vi "UHR-Fleezers Control (host) -TL FB Corrected Ronen semipassive - stepping.vi"(0 "Tab Control":T5(tab)=enum."Trap Control (RF)") -> ()   [LabVIEW 2013] (continued)
        n1835 = Build Array (concatenate)(w2860, w2859) -> (w2841:dbl[])
        n1836 = feedback #13(w2764) -> (w2766:dbl[])
        n1837 = Build Array (concatenate)(w2766, w2764) -> (w2765:dbl[])
        n1838 = local read "Scan steps (MCL)"() -> (w2746:u64)
        n1839 = Select(t=w2859, s=w2763, f=w2841) -> (s? t:f=w2845:dbl[])
        n1840 = feedback-in #12(w2845) -> ()
        n1841 = Select(t=w2764, s=w2763, f=w2765) -> (s? t:f=w2747:dbl[])
        n1842 = feedback-in #13(w2747) -> ()
        n1843 = local read "Scan lines (y)"() -> (w2732:u64)
        n1844 = local read "N APD Samp/step"() -> (w2748:dbl)
        n1845 = feedback #14(w2790) -> (w2847:dbl[])
        n1846 = Build Array (concatenate)(w2847, w2790) -> (w2838:dbl[])
        n1847 = feedback #15(w2797) -> (w2857:dbl[])
        n1848 = Build Array (concatenate)(w2857, w2797) -> (w2856:dbl[])
        n1849 = feedback #16(w2792) -> (w2849:dbl[])
        n1850 = Build Array (concatenate)(w2849, w2792) -> (w2850:dbl[])
        n1851 = Select(t=w2790, s=w2763, f=w2838) -> (s? t:f=w2794:dbl[])
        n1852 = feedback-in #14(w2794) -> ()
        n1853 = Select(t=w2797, s=w2763, f=w2856) -> (s? t:f=w2796:dbl[])
        n1854 = feedback-in #15(w2796) -> ()
        n1855 = Select(t=w2792, s=w2763, f=w2850) -> (s? t:f=w2795:dbl[])
        n1856 = feedback-in #16(w2795) -> ()
        n1857 = Multiply(x=w2746, y=u64 2) -> (x*y=w2731:u64)
        n1858 = call "integrate 1D array interval - double.vi"("Ave N"=w2748, "Array In"=w2747) -> ("Array Out"=w2759:dbl[])  [unwired: 1 out]
        n1859 = call "integrate 1D array interval - double.vi"("Ave N"=w2748, "Array In"=w2845) -> ("Array Out"=w2844:dbl[])  [unwired: 1 out]
        n1860 = Array Size(array=w2759) -> (size(s)=w2760:i32)
        n1861 = Array Size(array=w2844) -> (size(s)=w2846:i32)
        n1862 = Multiply(x=w2732, y=w2731) -> (x*y=w2762:u64)
        n1863 = Multiply(x=w2732, y=w2731) -> (x*y=w2854:u64)
        n1864 = call-poly <vilib>:"Mean.vi"("X"=w2794) -> ("mean"=w2778:dbl)  [unwired: 1 out]
        n1865 = Subtract(x=w2762, y=w2760) -> (x-y=w2753:u64)
        n1866 = call-poly <vilib>:"Mean.vi"("X"=w2796) -> ("mean"=w2783:dbl)  [unwired: 1 out]
        n1867 = call-poly <vilib>:"Mean.vi"("X"=w2795) -> ("mean"=w2781:dbl)  [unwired: 1 out]
        n1868 = call-poly <vilib>:"Mean.vi"("X"=w2759) -> ("mean"=w2750:dbl)  [unwired: 1 out]
        n1869 = Subtract(x=w2854, y=w2846) -> (x-y=w2788:u64)
        n1870 = call-poly <vilib>:"Mean.vi"("X"=w2844) -> ("mean"=w2785:dbl)  [unwired: 1 out]
        n1871 = Initialize Array(1.0 ("element"), w2753) -> (w2749:dbl[])
        n1872 = Initialize Array(1.0 ("element"), w2788) -> (w2779:dbl[])
        n1873 = Multiply(x=w2749, y=w2750) -> (x*y=w2751:dbl[])
        n1874 = Multiply(x=w2779, y=w2781) -> (x*y=w2782:dbl[])
        n1875 = Multiply(x=w2779, y=w2783) -> (x*y=w2784:dbl[])
        n1876 = Multiply(x=w2779, y=w2778) -> (x*y=w2780:dbl[])
        n1877 = Multiply(x=w2779, y=w2785) -> (x*y=w2786:dbl[])
        n1878 = Build Array (concatenate)(w2794, w2780) -> (w2848:dbl[])
        n1879 = Build Array (concatenate)(w2796, w2784) -> (w2852:dbl[])
        n1880 = Build Array (concatenate)(w2795, w2782) -> (w2851:dbl[])
        n1881 = Build Array (concatenate)(w2759, w2751) -> (w2761:dbl[])
        n1882 = Build Array (concatenate)(w2844, w2786) -> (w2853:dbl[])
        n1883 = Reshape Array(w2848, w2732, w2731) -> (w2814:dbl[][])
        n1884 = Reshape Array(w2761, w2732, w2731) -> (w2757:dbl[][])
        n1885 = Reshape Array(w2852, w2732, w2731) -> (w2806:dbl[][])
        n1886 = Reshape Array(w2851, w2732, w2731) -> (w2821:dbl[][])
        n1887 = Reshape Array(w2853, w2732, w2731) -> (w2831:dbl[][])
        n1888 = Array Subset(array=w2821, index (col)=0 ("index"), length (col)=w2746) -> (w2826:dbl[][])  [unwired: 2 in]
        n1889 = Array Subset(array=w2821, index (col)=w2746) -> (w2824:dbl[][])  [unwired: 3 in]
        n1890 = Array Subset(array=w2806, index (col)=0 ("index"), length (col)=w2746) -> (w2812:dbl[][])  [unwired: 2 in]
        n1891 = Array Subset(array=w2806, index (col)=w2746) -> (w2810:dbl[][])  [unwired: 3 in]
        n1892 = Array Subset(array=w2757, index (col)=0 ("index"), length (col)=w2746) -> (w2756:dbl[][])  [unwired: 2 in]
        n1893 = Array Subset(array=w2757, index (col)=w2746) -> (w2754:dbl[][])  [unwired: 3 in]
        n1894 = Array Subset(array=w2831, index (col)=0 ("index"), length (col)=w2746) -> (w2830:dbl[][])  [unwired: 2 in]
        n1895 = Array Subset(array=w2831, index (col)=w2746) -> (w2828:dbl[][])  [unwired: 3 in]
        n1896 = Array Subset(array=w2814, index (col)=0 ("index"), length (col)=w2746) -> (w2819:dbl[][])  [unwired: 2 in]
        n1897 = Array Subset(array=w2814, index (col)=w2746) -> (w2817:dbl[][])  [unwired: 3 in]
        n1898 = for {
          tunnel: w2826 -> [w2868] mode=indexing
          tunnel: [w2867] -> w2825 mode=indexing
          workers-P: _ -> [_]
          n1899 = Reverse 1D Array(array=w2868) -> (reversed array=w2867:dbl[])
        }
        n1900 = for {
          tunnel: w2812 -> [w2864] mode=indexing
          tunnel: [w2863] -> w2811 mode=indexing
          workers-P: _ -> [_]
          n1901 = Reverse 1D Array(array=w2864) -> (reversed array=w2863:dbl[])
        }
        n1902 = for {
          tunnel: w2756 -> [w2862] mode=indexing
          tunnel: [w2861] -> w2755 mode=indexing
          workers-P: _ -> [_]
          n1903 = Reverse 1D Array(array=w2862) -> (reversed array=w2861:dbl[])
        }
        n1904 = for {
          tunnel: w2830 -> [w2870] mode=indexing
          tunnel: [w2869] -> w2829 mode=indexing
          workers-P: _ -> [_]
          n1905 = Reverse 1D Array(array=w2870) -> (reversed array=w2869:dbl[])
        }
        n1906 = for {
          tunnel: w2819 -> [w2866] mode=indexing
          tunnel: [w2865] -> w2818 mode=indexing
          workers-P: _ -> [_]
          n1907 = Reverse 1D Array(array=w2866) -> (reversed array=w2865:dbl[])
        }
        n1908 = Index Array(array=w2831, index (row)=0) -> (element=→"Waveform Graph":dbl[])  [unwired: 1 in]
        n1909 = Add(x=w2825, y=w2824) -> (x+y=w2823:dbl[][])
        n1910 = Add(x=w2811, y=w2810) -> (x+y=w2809:dbl[][])
        n1911 = Add(x=w2755, y=w2754) -> (x+y=w2739:dbl[][])
        n1912 = Add(x=w2829, y=w2828) -> (x+y=w2803:dbl[][])
        n1913 = Add(x=w2818, y=w2817) -> (x+y=w2816:dbl[][])
        n1914 = Divide(x=w2809, y=2) -> (x/y=w2807:dbl[][])
        n1915 = Divide(x=w2823, y=2) -> (x/y=w2768:dbl[][])
        n1916 = Divide(x=w2816, y=2) -> (x/y=w2770:dbl[][])
        n1917 = To Single Precision Float(number=w2803) -> (single precision float=w2802:sgl[][])
        n1918 = Transpose 2D Array(2D array=w2807) -> (transposed array=→"Data map":dbl[][])
        n1919 = To Single Precision Float(number=w2739) -> (single precision float=w2743:sgl[][])
        n1920 = To Single Precision Float(number=w2768) -> (single precision float=w2774:sgl[][])
        n1921 = To Single Precision Float(number=w2770) -> (single precision float=w2771:sgl[][])
        n1922 = call "IMAQ ArrayToImage"("Image Pixels (Float)"=w2802, "Image"=w2736) -> ("Image Out"=w2805:T3)  [unwired: 8 in, 1 out]
        n1923 = call "IMAQ ArrayToImage"("Image Pixels (Float)"=w2743, "Image"=w2735) -> ("Image Out"=w2745:T3)  [unwired: 8 in, 1 out]
        n1924 = call "IMAQ ArrayToImage"("Image Pixels (Float)"=w2774, "Image"=w2734) -> ("Image Out"=w2776:T3)  [unwired: 8 in, 1 out]
        n1925 = call "IMAQ ArrayToImage"("Image Pixels (Float)"=w2771, "Image"=w2733) -> ("Image Out"=w2773:T3)  [unwired: 8 in, 1 out]
        n1926 = call "IMAQ Symmetry"("Type of Symmetry"=w2804, "Image Src"=w2805) -> ("Image Dst Out"=w2800:T3)  [unwired: 3 in, 1 out]
        n1927 = call "IMAQ Symmetry"("Type of Symmetry"=w2744, "Image Src"=w2745) -> ("Image Dst Out"=w2741:T3)  [unwired: 3 in, 1 out]
        n1928 = call "IMAQ Symmetry"("Type of Symmetry"=w2775, "Image Src"=w2776) -> ("Image Dst Out"=→"Detection Laser X":T3)  [unwired: 3 in, 1 out]
        n1929 = call "IMAQ Symmetry"("Type of Symmetry"=w2772, "Image Src"=w2773) -> ("Image Dst Out"=→"Detection Laser Y":T3)  [unwired: 3 in, 1 out]
        n1930 = call "IMAQ Set Simple Calibration"("Calibration Axis Info"=T37 {"Origin Pixel"={"X"=0.0, "Y"=0.0}, "Angle Relative to Horizontal (deg)"=0.0, "Axis Reference"=0}, "Grid Descriptor"=T38 {"X Step"=0.3, "Y Step"=0.3, "Unit"=enum."Undefined"}, "Image"=w2800) -> ("Calibrated Image"=→"APD 1":T3)  [unwired: 7 in, 1 out]
        n1931 = call "IMAQ Set Simple Calibration"("Calibration Axis Info"=T37 {"Origin Pixel"={"X"=0.0, "Y"=0.0}, "Angle Relative to Horizontal (deg)"=0.0, "Axis Reference"=0}, "Grid Descriptor"=T38 {"X Step"=0.3, "Y Step"=0.3, "Unit"=enum."Undefined"}, "Image"=w2741) -> ("Calibrated Image"=→"APD 2":T3)  [unwired: 7 in, 1 out]
      }
    }
    n1932 = Subtract(x=w2283, y="APD 2 Offset") -> (x-y=w2280:waveform(dbl))
    n1933 = Subtract(x=w2285, y="APD 1 Offset") -> (x-y=w2281:waveform(dbl))
    n1934 = Index Array(array=w2300, index=3) -> (element=w2367:waveform(dbl))
    n1935 = Index Array(array=w2300, index=6) -> (element=w2364:waveform(dbl))
    n1936 = Build Array(w2281, w2280) -> (→"APD Chart":waveform(dbl)[])
    n1937 = Array Size(array=w2357) -> (size(s)=w2407:i32)
    n1938 = call <vilib>:"Std Deviation and Variance.vi"("X"=w2293) -> ("standard deviation"=w2292:dbl)  [unwired: 1 in, 2 out]
    n1939 = Add Array Elements(numeric array=w2293) -> (sum=w2295:u32)
    n1940 = Add Array Elements(numeric array=w2357) -> (sum=w2417:u32)
    n1941 = call <vilib>:"Std Deviation and Variance.vi"("X"=w2357) -> ("standard deviation"=w2356:dbl)  [unwired: 1 in, 2 out]
    n1942 = Divide(x=w2292, y=w2291) -> (x/y=w2288:dbl)
    "Rate sigma (Hz) 2" <- w2288
    n1943 = Multiply(x=w2291, y=w2407) -> (x*y=w2294:dbl)
    "Int. Time (s)" <- w2294
    n1944 = Divide(x=w2295, y=w2294) -> (x/y=w2289:dbl)
    "APD 2 Rate (Hz)" <- w2289
    n1945 = Divide(x=w2417, y=w2294) -> (x/y=w2354:dbl)
    "APD 1 Rate (Hz)" <- w2354
    n1946 = Divide(x=w2356, y=w2291) -> (x/y=w2355:dbl)
    "Rate sigma (Hz)" <- w2355
    n1947 = Divide(x=w2288, y=w2289) -> (x/y=→"Sigma/Mean 2":dbl)
    n1948 = Divide(x=w2355, y=w2354) -> (x/y=→"Sigma/Mean":dbl)
    n1949 = case shown="2" "Calibration" {
      tunnel: "T1 alpha_x (nm/V)" -> [_ w2699 w2720]
      tunnel: "T1 kappa_x (pN/nm)" -> [_ _ w2710]
      tunnel: "T2 alpha_x (nm/V)" -> [_ w2698 w2718]
      tunnel: "T2 kappa_x (pN/nm)" -> [_ _ w2711]
      tunnel: w2367 -> [w2681 w2696 w2716]
      tunnel: w2364 -> [w2680 w2694 w2714]
      tunnel: [w2681 w2693 w2713] -> w2393
      tunnel: [w2680 w2692 w2712] -> w2392
      tunnel: ["T1 X (V)" ("Label.Text") "T1 X (nm)" ("Label.Text") "T1 X (pN)" ("Label.Text")] -> w2385
      tunnel: ["T2 X (V)" ("Label.Text") "T2 X (nm)" ("Label.Text") "T2 X (pN)" ("Label.Text")] -> w2384
      tunnel: ["Position (V)" ("Label.Text") "Position (nm)" ("Label.Text") "Force (pN)" ("Label.Text")] -> w2386
      tunnel: w2366 -> [_ w2684 w2703]
      tunnel: w2368 -> [_ w2687 w2705]
      tunnel: ["Mean (V)" ("Label.Text") "Mean (nm)" ("Label.Text") "Mean (pN)" ("Label.Text")] -> w2381
      tunnel: ["Difference (V)" ("Label.Text") "Difference (nm)" ("Label.Text") "Difference (pN)" ("Label.Text")] -> w2308
      frame 0, Default {
      }
      frame 1 {
        # "position"
        n1950 = Unbundle By Name(w2696) -> ("Y"=w2700:dbl[])
        n1951 = Unbundle By Name(w2694) -> ("Y"=w2685:dbl[])
        n1952 = Subtract(x=w2700, y=w2687) -> (x-y=w2688:dbl[])
        n1953 = Subtract(x=w2685, y=w2684) -> (x-y=w2686:dbl[])
        n1954 = Multiply(x=w2686, y=w2698) -> (x*y=w2695:dbl[])
        n1955 = Multiply(x=w2699, y=w2688) -> (x*y=w2697:dbl[])
        n1956 = Bundle By Name(cluster=w2694, "Y"=w2695) -> (w2692:waveform(dbl))
        n1957 = Bundle By Name(cluster=w2696, "Y"=w2697) -> (w2693:waveform(dbl))
      }
      frame 2 {
        # "force"
        n1958 = Unbundle By Name(w2716) -> ("Y"=w2721:dbl[])
        n1959 = Unbundle By Name(w2714) -> ("Y"=w2719:dbl[])
        n1960 = Subtract(x=w2719, y=w2703) -> (x-y=w2704:dbl[])
        n1961 = Subtract(x=w2721, y=w2705) -> (x-y=w2706:dbl[])
        n1962 = Compound Arithmetic op=MULTIPLY(w2704, w2718, w2711) -> (w2715:dbl[])
        n1963 = Compound Arithmetic op=MULTIPLY(w2710, w2720, w2706) -> (w2717:dbl[])
        n1964 = Bundle By Name(cluster=w2714, "Y"=w2715) -> (w2712:waveform(dbl))
        n1965 = Bundle By Name(cluster=w2716, "Y"=w2717) -> (w2713:waveform(dbl))
      }
    }
    n1966 = feedback-in #17("Calibration") -> ()
    n1967 = feedback #17(u16 1 ("Calibration")) -> (w2388:u16)
    n1968 = local read "Trap 2 Bead Size (nm)"() -> (w2188:dbl)
    n1969 = local read "Trap 1 Bead Size (nm)"() -> (w2187:dbl)
    n1970 = local read "AOM X Cal (nm/MHz)"() -> (w2185:dbl)
    n1971 = local read "Trap Delta (MHz)"() -> (w2184:dbl)
    n1972 = Not Equal?(x=w2388, y="Calibration") -> (x != y?=w2345:bool)
    n1973 = Multiply(x=w2185, y=w2184) -> (x*y=w2189:dbl)
    n1974 = Add(x=w2188, y=w2187) -> (x+y=w2191:dbl)
    n1975 = Unbundle By Name(w2367) -> ("Y"=w2370:dbl[])
    n1976 = Unbundle By Name(w2364) -> ("Y"=w2373:dbl[])
    n1977 = Divide(x=w2191, y=2.0) -> (x/y=w2186:dbl)
    n1978 = Subtract(x=w2370, y=w2368) -> (x-y=w2371:dbl[])
    n1979 = Subtract(x=w2373, y=w2366) -> (x-y=w2372:dbl[])
    n1980 = disable-structure shown="Enabled" {
      disable-tunnel: [-1.0 ("y") 1.0] -> w2374
      frame Disabled {
      }
      frame Enabled {
      }
    }
    n1981 = Multiply(x=w2372, y="T2 alpha_x (nm/V)") -> (x*y=w2363:dbl[])
    n1982 = Multiply(x="T1 alpha_x (nm/V)", y=w2371) -> (x*y=w2362:dbl[])
    n1983 = Multiply(x=w2392, y=w2374) -> (x*y=w2375:waveform(dbl))
    n1984 = case shown="False" "Read Lateness and Rel Phase" {
      tunnel: w2161 -> [w2647 w2669]
      tunnel: w2200 -> [w2648 w2668]
      tunnel: [w2647 w2667] -> w2360
      tunnel: [w2648 w2666] -> w2359
      frame False {
      }
      frame True {
        n1985 = xnode "Read/Write Control"("FPGA VI Reference In"=w2669, "error in"=w2668) -> ("FPGA VI Reference Out"=w2667:T20, "error out"=w2666:errorcluster, "GI Relative phase"=→"GI relative phase":i16, "Relative phase"=→"Relative phase (AI1)":i16, "AI Late Counter"=→"Late Counter (AI1)":u8, "GI Late Counter"=→"GI Late Counter":u8, "MCL Late Counter"=→"MCL Late Counter":u8, "MCL Relative Phase"=→"Relative Phase (MCL)":i16, "APD Acq Relative Phase"=→"APD Acq Relative Phase":i16, "APD 1 Gate Relative Phase"=→"APD 1 Gate Relative Phase":i16, "APD 2 Gate Relative Phase"=→"APD 2 Gate Relative Phase":i16, "APD Acq Late Counter"=→"APD Acq Late Counter":u16, "APD 1 Gate Late Counter"=→"APD 1 Gate Late Counter":u8, "APD 2 Gate Late Counter"=→"APD 2 Gate Late Counter":u8, "Green FB Relative Phase"=→"Relative phase (Green FB)":i16, "GI Relative phase 2"=→"GI relative phase 2":i16, "GI Late Counter 2"=→"GI Late Counter 2":u16, "Trap Pos FIFO Timeout"=→"Trap Pos FIFO Timeout":u16, "Trap AI FIFO Timeout"=→"Trap AI FIFO Timeout":u16)
      }
    }
    n1986 = Subtract(x=w2363, y=w2362) -> (x-y=w2183:dbl[])
    n1987 = call-poly <vilib>:"Mean.vi"("X"=w2183) -> ("mean"=w2190:dbl)  [unwired: 1 out]
    n1988 = Add(x=w2189, y=w2190) -> (x+y=w2193:dbl)
    n1989 = Subtract(x=w2193, y=w2186) -> (x-y=→"Tether Extension (nm, calculated)":dbl)
    n1990 = Unbundle By Name(w2392) -> ("Y"=w2333:dbl[])
    n1991 = Unbundle By Name(w2393) -> ("Y"=w2334:dbl[])
    n1992 = Build Array(w2393, w2375) -> (→"Force":waveform(dbl)[])
    n1993 = Subtract(x=w2183, y="Offset (nm)") -> (x-y=w2331:dbl[])
    n1994 = call-poly <vilib>:"Mean.vi"("X"=w2333) -> ("mean"=w2312:dbl)  [unwired: 1 out]
    "T2 X" <- w2312
    n1995 = Absolute Value(x=w2334) -> (abs(x)=w2335:dbl[])
    n1996 = Absolute Value(x=w2333) -> (abs(x)=w2336:dbl[])
    n1997 = call-poly <vilib>:"Mean.vi"("X"=w2334) -> ("mean"=w2313:dbl)  [unwired: 1 out]
    "T1 X" <- w2313
    n1998 = Add(x=w2335, y=w2336) -> (x+y=w2337:dbl[])
    n1999 = Bundle By Name(cluster=w2367, "Y"=w2331) -> (w2299:waveform(dbl))
    "Bead Separation" <- w2299
    n2000 = Divide(x=w2337, y=2.0) -> (x/y=→"Vec Mean of T1 T2":dbl[])
    n2001 = case shown="True" w2345 {
      tunnel: w2386 -> [_ w2674]
      tunnel: w2385 -> [_ w2673]
      tunnel: w2384 -> [_ w2672]
      tunnel: w2381 -> [_ w2671]
      tunnel: w2308 -> [_ w2670]
      frame False {
      }
      frame True {
        n2002 = property on="Force" class="WFChart (strict)"("YScale.NameLbl.Text"=w2674) -> ()  [unwired: 2 in, 2 out]
        n2003 = property on="T2 X" class="DigNum (strict)"("Caption.Text"=w2672) -> ()  [unwired: 2 in, 2 out]
        n2004 = property on="T1 X" class="DigNum (strict)"("Caption.Text"=w2673) -> ()  [unwired: 2 in, 2 out]
        n2005 = property on="Mean" class="DigNum (strict)"("Caption.Text"=w2671) -> ()  [unwired: 2 in, 2 out]
        n2006 = property on="Difference" class="DigNum (strict)"("Caption.Text"=w2670) -> ()  [unwired: 2 in, 2 out]
      }
    }
    n2007 = local read "Tether"() -> (w2339:bool)
    n2008 = Absolute Value(x=w2313) -> (abs(x)=w2310:dbl)
    n2009 = Absolute Value(x=w2312) -> (abs(x)=w2309:dbl)
    n2010 = Add(x=w2310, y=w2309) -> (x+y=w2383:dbl)
    n2011 = Subtract(x=w2310, y=w2309) -> (x-y=→"Difference":dbl)
    n2012 = feedback #18(w2331) -> (w2330:dbl[])
    n2013 = Divide(x=w2383, y=2.0) -> (x/y=w2158:dbl)
    "Mean" <- w2158
    n2014 = case shown="True" w2339 {
      tunnel: w2158 -> [_ w2606]
      frame False {
      }
      frame True {
        n2015 = Greater?(x="Lost Tether Alarm Threshold (pN)", y=w2606) -> (0:w2604:bool)
        n2016 = case shown="True" w2604 {
          frame False {
          }
          frame True {
            n2017 = flat-sequence {
              frame #0 {
                # "stop only if saving"
                n2018 = local read "Saving..."() -> (w2619:bool)
                n2019 = And(x=w2619, y="TA Cancel Save?") -> (x .and. y?=w2618:bool)
                n2020 = local write "Stop Saving"(w2618) -> ()
              }
              frame #1 {
                n2021 = case shown="True" "TA Green Off?" {
                  frame False {
                  }
                  frame True {
                    w2622 = FALSE ("Fl. Triggered...")
                    n2022 = local write "Fl. Triggered..."(w2622) -> ()
                    n2023 = property on="Green Laser ON/Interlacing" class="Bool (strict)"("Val(Sgnl)"=w2622) -> ()  [unwired: 2 in, 2 out]
                  }
                }
              }
            }
            n2024 = local read "Time tether formed"() -> (w2613:timestamp)
            n2025 = Get Date/Time In Seconds() -> (seconds since 1Jan1904=w2614:timestamp)
            n2026 = Subtract(x=w2614, y=w2613) -> (x-y=w2612:dbl)
            n2027 = Number To Decimal String(number=w2612) -> (decimal integer string=w2609:string)  [unwired: 1 out]
            n2028 = local read "Messages"() -> (w2616:string)
            n2029 = call <vilib>:"Beep.vi"() -> ()  [unwired: 3 in, 9 out]
            n2030 = Concatenate Strings("Lost tether (" ("Message to add"), w2609, " s)." ("string")) -> (w2611:string)
            n2031 = local write "Tether"(FALSE ("Tether")) -> ()
            n2032 = call "Update messages.vi"("Message to add"=w2611, "Old message string"=w2616) -> ("New message string"=w2615:string)
            n2033 = local write "Messages"(w2615) -> ()
            n2034 = property on="Trap Pos. FB ON" class="Bool (strict)"("Val(Sgnl)"=FALSE ("Value (Signaling)")) -> ()  [unwired: 2 in, 2 out]
          }
        }
      }
    }
    n2035 = Build Array (concatenate)(w2331, w2330) -> (w2329:dbl[])
    n2036 = Split 1D Array(array=w2329, index=w2211) -> (first subarray=w2325:dbl[])  [unwired: 1 out]
    n2037 = feedback-in #18(w2325) -> ()
    n2038 = call-poly <vilib>:"Mean.vi"("X"=w2325) -> ("mean"=w2324:dbl)  [unwired: 1 out]
    "Bead Mean (nm)" <- w2324
    n2039 = Subtract(x=w2325, y=w2324) -> (x-y=w2323:dbl[])
    n2040 = Square(x=w2323) -> (x^2=w2322:dbl[])
    n2041 = case shown="True" "Semi Passive ON" {
      tunnel: "Semi Passive mode" -> [_ w2485]
      tunnel: "Jump Force (pN)" -> [_ w2484]
      tunnel: w2158 -> [_ w2483]
      frame False {
      }
      frame True {
        n2042 = case shown="\"Use Feedback\"" w2485 {
          tunnel: w2484 -> [_ w2488 w2504]
          tunnel: w2483 -> [_ w2487 w2503]
          frame "None" {
          }
          frame "Use Feedback" {
            n2043 = local read "Target Force (pN)"() -> (w2490:dbl)
            n2044 = Less?(x=w2488, y=w2490) -> (x < y?=w2489:bool)
            n2045 = case shown="True" w2489 {
              tunnel: w2488 -> [w2497 w2500]
              tunnel: w2487 -> [w2496 w2499]
              tunnel: [w2495 w2498] -> w2486
              frame False {
                n2046 = Less?(x=w2497, y=w2496) -> (x < y?=w2495:bool)
              }
              frame True {
                n2047 = Greater?(x=w2500, y=w2499) -> (0:w2498:bool)
              }
            }
            n2048 = case shown="True" w2486 {
              frame False {
                n2049 = local read "Trap Pos. FB ON"() -> (w2491:bool)
                n2050 = case shown="True" w2491 {
                  frame False {
                  }
                  frame True {
                    n2051 = property on="Trap Pos. FB ON" class="Bool (strict)"("Val(Sgnl)"=FALSE) -> ()  [unwired: 2 in, 2 out]
                  }
                }
              }
              frame True {
                n2052 = local read "Trap Pos. FB ON"() -> (w2493:bool)
                n2053 = case shown="False" w2493 {
                  frame False {
                    n2054 = property on="Trap Pos. FB ON" class="Bool (strict)"("Val(Sgnl)"=TRUE) -> ()  [unwired: 2 in, 2 out]
                  }
                  frame True {
                  }
                }
              }
            }
          }
          frame "Sharp Jump" {
            n2055 = local read "Target Force (pN)"() -> (w2506:dbl)
            n2056 = Greater?(x=w2504, y=w2506) -> (0:w2505:bool)
            n2057 = case shown="True" w2505 {
              tunnel: w2504 -> [w2521 w2525]
              tunnel: w2503 -> [w2522 w2524]
              tunnel: [w2520 w2523] -> w2502
              frame False {
                n2058 = Greater?(x=w2522, y=w2521) -> (0:w2520:bool)
              }
              frame True {
                n2059 = Less?(x=w2525, y=w2524) -> (x < y?=w2523:bool)
              }
            }
            n2060 = Subtract(x=w2504, y=w2506) -> (x-y=w2501:dbl)
            n2061 = case shown="True" w2502 {
              tunnel: w2501 -> [_ w2512]
              frame False {
              }
              frame True {
                n2062 = local read "T1 kappa_x (pN/nm)"() -> (w2517:dbl)
                n2063 = local read "T2 kappa_x (pN/nm)"() -> (w2518:dbl)
                n2064 = Reciprocal(x="DNA stiffness (pN / nm)") -> (1/x=w2514:dbl)
                n2065 = Reciprocal(x=w2517) -> (1/x=w2516:dbl)
                n2066 = Reciprocal(x=w2518) -> (1/x=w2515:dbl)
                n2067 = Compound Arithmetic op=ADD(w2516, w2515, w2514) -> (w2513:dbl)
                n2068 = local read "AOM X Cal (nm/MHz)"() -> (w2511:dbl)
                n2069 = Multiply(x=w2513, y=w2512) -> (x*y=w2510:dbl)
                n2070 = local read "Trap Delta (MHz)"() -> (w2508:dbl)
                n2071 = Divide(x=w2510, y=w2511) -> (x/y=w2509:dbl)
                n2072 = Subtract(x=w2508, y=w2509) -> (x-y=w2507:dbl)
                n2073 = property on="Trap Delta (MHz)" class="DigNum (strict)"("Val(Sgnl)"=w2507) -> ()  [unwired: 2 in, 2 out]
              }
            }
          }
        }
      }
    }
    n2074 = call-poly <vilib>:"Mean.vi"("X"=w2322) -> ("mean"=w2321:dbl)  [unwired: 1 out]
    n2075 = Square Root(x=w2321) -> (sqrt(x)=w2320:dbl)
    n2076 = Multiply(x=10.0, y=w2320) -> (x*y=→"RMS (Ang)":dbl)
    n2077 = xnode "Read/Write Control"("FPGA VI Reference In"=w2360, "error in"=w2359) -> ("FPGA VI Reference Out"=w2471:T20, "error out"=w2465:errorcluster, "AI4 Y Sum Set 1"=w2461, "AI4 Y Sum Set 2"=w2460, "AI1 X Set 1"=w2245:fxp<+/-,16,1>, "AI1 X Set 2"=w2244:fxp<+/-,16,1>, "Trap Pos FB Int Signal"=→"Trap Pos FB Int Signal":fxp<+/-,24,9>, "Trap Pos FB Int-Norm Signal"=→"Trap Pos FB Int-Norm Signal":fxp<+/-,16,1>, "Trap Pos FB Action"=w2238:i64, "Scanning"=→"AOD Scanning":bool, "Scan I"=→"AOD Scan I":u64, "Scanning MCL"=w2463:bool, "Scan I (MCL)"=→"MCL Scan I":u64, "Green FB Signals"=w2402:T48)  [unwired: 1 out]
    "MCL Scanning" <- w2463
    "Trap Pos FB Action" <- w2238
    n2078 = local read "AI2 (V)"() -> (w2462:cluster{"Set 1":dbl, "Set 2":dbl})
    n2079 = Bundle By Name(cluster=w2462, "Set 1"=w2461, "Set 2"=w2460) -> (w2458:cluster{"Set 1":dbl, "Set 2":dbl})
    n2080 = Divide(x=w2238, y=327.67) -> (x/y=→"Action (%)":dbl)
    n2081 = local read "Trap X (AI1)"() -> (w2258:T1)
    n2082 = Divide(x=w2458, y=3276.7) -> (x/y=w2457:cluster{"Set 1":dbl, "Set 2":dbl})
    n2083 = local write "AI2 (V)"(w2457) -> ()
    n2084 = Bundle(cluster=w2258, "Trap 1"=w2245, "Trap 2"=w2244) -> (→"Trap X (AI1)":T1)
    n2085 = Divide(x=w2402, y=3276.7) -> (x/y=w2398:T49)
    n2086 = Unbundle By Name(w2398) -> ("Green FB Ch 0"=w2401:dbl, "Green FB Ch 1"=w2400:dbl, "Green FB Ch 2"=w2399:dbl)
    n2087 = Divide(x=w2401, y=w2399) -> (x/y=w2397:dbl)
    n2088 = Divide(x=w2400, y=w2399) -> (x/y=w2396:dbl)
    n2089 = flat-sequence "To save data" {
      tunnel: [w3496] -> w2482
      tunnel: [w3497] -> w2481
      tunnel: w2433 -> [w3490]
      tunnel: w2327 -> [w3494]
      tunnel: ["Save Calibration"] -> w2454
      tunnel: w2451 -> [w3493]
      tunnel: [w3486] -> w2450
      tunnel: [w3483] -> w2449
      tunnel: [w3480] -> w2448
      tunnel: w2432 -> [w3482]
      tunnel: w2343 -> [w3476]
      tunnel: [w3476] -> w2342
      tunnel: ["Start Saving"] -> w2301
      tunnel: [w3470] -> w2227
      tunnel: [w3469] -> w2226
      tunnel: w2482 -> [w3731]
      tunnel: w2481 -> [w3730]
      tunnel: w2228 -> [w3729]
      tunnel: w2454 -> [w3728]
      tunnel: w2450 -> [w3726]
      tunnel: w2449 -> [w3725]
      tunnel: w2448 -> [w3724]
      tunnel: w2314 -> [w3723]
      tunnel: w2352 -> [w3722]
      tunnel: w2342 -> [w3721]
      tunnel: w2301 -> [w3720]
      tunnel: w2299 -> [w3719]
      tunnel: w2275 -> [w3718]
      tunnel: w2227 -> [w3717]
      tunnel: w2226 -> [w3716]
      tunnel: w2225 -> [w3715]
      frame #0 {
        n2090 = Or(x="Save N Sets", y="Start Saving") -> (x .or. y?=w3477:bool)
        n2091 = To Double Precision Float(number=w3493) -> (double precision float=w3487:dbl)
        n2092 = Build Array(w3477, "Save Calibration", w3490, w3482) -> (w3492:bool[])
        n2093 = Compound Arithmetic op=OR("Save Calibration", w3490, w3477, w3482) -> (w3495:bool)
        n2094 = Boolean Array To Number(Boolean array=w3492) -> (number=w3489:u32)
        n2095 = feedback #19(FALSE ("Save APD Data\nwith Trap Data")) -> (w3471:bool)
        n2096 = feedback #20(refnum<k0> refnum) -> (w3498:refnum<file>)
        n2097 = feedback #21(refnum<k0> refnum) -> (w3473:refnum<file>)
        n2098 = feedback #22(FALSE ("Save APD Data\nwith Trap Data")) -> (w3481:bool)
        n2099 = feedback #23(refnum<k0> refnum) -> (w3484:refnum<file>)
        n2100 = feedback #24(0) -> (w3500:i32)
        n2101 = feedback #25() -> (w3488:u32)  [unwired: 1 out]
        n2102 = case shown="True" w3495 {
          tunnel: [w3507 1] -> w3496
          tunnel: w3500 -> [w3509 _]
          tunnel: [w3508 w3527] -> w3497
          tunnel: w3498 -> [w3508 _]
          tunnel: w3494 -> [_ w3547]
          tunnel: w3487 -> [_ w3545]
          tunnel: w3489 -> [_ w3548]
          tunnel: [w3506 w3526] -> w3486
          tunnel: w3488 -> [w3506 _]
          tunnel: [w3505 w3524] -> w3483
          tunnel: w3484 -> [w3505 _]
          tunnel: [w3504 w3523] -> w3480
          tunnel: w3481 -> [w3504 _]
          tunnel: "Start Saving" -> [_ w3521]
          tunnel: w3476 -> [_ w3520]
          tunnel: [w3503 w3511] -> w3469
          tunnel: w3473 -> [w3503 _]
          tunnel: [w3502 w3510] -> w3470
          tunnel: w3471 -> [w3502 _]
          frame False {
            n2103 = Increment(x=w3509) -> (x+1=w3507:i32)
          }
          frame True {
            w3517 = FALSE ("Start Saving")
            w3522 = 9.0  # File Version
            w3530 = FALSE ("prepend array or string size? (T)")
            w3528 = T30."big-endian, network order" ("byte order (0:big-endian, network order)")
            # "write file headers"
            n2104 = local read "BD 1 Frequency 1 (MHz)"() -> (w3544:dbl)
            n2105 = local read "BD 2 Frequency 1 (MHz)"() -> (w3543:dbl)
            n2106 = local read "BD 1 Frequency 2 (MHz)"() -> (w3542:dbl)
            n2107 = local read "BD 2 Frequency 2 (MHz)"() -> (w3541:dbl)
            n2108 = local read "BD 1 Frequency 3 (MHz)"() -> (w3540:dbl)
            n2109 = local read "BD 2 Frequency 3 (MHz)"() -> (w3539:dbl)
            n2110 = Array Size(array=w3520) -> (size(s)=w3519:i32)
            n2111 = To Double Precision Float(number=w3519) -> (double precision float=w3518:dbl)
            n2112 = local write "Save Calibration"(w3517) -> ()
            n2113 = local write "Start Saving"(w3517) -> ()
            n2114 = Build Array("Save APD Data\nwith Trap Data", "Save Trap Pos. Data") -> (w3514:bool[])
            n2115 = Boolean Array To Number(Boolean array=w3514) -> (number=w3513:u32)
            n2116 = Build Array(w3544, w3543, w3542, w3541, w3540, w3539) -> (w3538:dbl[])
            n2117 = case shown="4" w3548 {
              tunnel: w3547 -> [w3619 w3639 w3655 w3693]
              tunnel: w3518 -> [w3624 w3646 w3675 w3712]
              tunnel: w3545 -> [w3623 w3645 w3674 w3711]
              tunnel: [w3620 w3641 w3666 w3703] -> w3536
              tunnel: [w3611 "Cal sets to save" w3656 w3694] -> w3526
              tunnel: w3538 -> [w3621 w3642 w3668 w3705]
              tunnel: "Save APD Data\nwith Trap Data" -> [w3618 _ w3652 w3691]
              tunnel: [w3618 w3633 w3652 w3691] -> w3523
              tunnel: w3522 -> [w3614 w3634 w3650 w3689]
              tunnel: w3521 -> [w3613 _ _ _]
              tunnel: [w3604 w3633 w3649 w3679] -> w3510
              tunnel: "Save Trap Pos. Data" -> [w3604 _ w3649 w3679]
              tunnel: w3513 -> [w3603 _ w3648 w3678]
              frame 1, Default {
                # "timeseries"
                n2118 = case shown="True" "Profile" {
                  tunnel: [w3627 w3630] -> w3608
                  tunnel: [w3627 w3629] -> w3607
                  tunnel: [w3627 w3628] -> w3606
                  tunnel: [w3627 w3632] -> w3605
                  frame False {
                    w3627 = 0.0 ("f")
                  }
                  frame True {
                    n2119 = local read "Current Position"() -> (w3631:dbl[])
                    n2120 = local read "Y change (mm)"() -> (w3632:dbl)
                    n2121 = call "subVI_explode3array.vi"("Array"=w3631) -> ("x"=w3630:dbl, "y"=w3629:dbl, "z"=w3628:dbl)  [unwired: 12 in]
                  }
                }
                n2122 = local read "Save ave N"() -> (w3626:dbl)
                n2123 = Multiply(x=w3626, y=w3619) -> (x*y=w3625:dbl)
                n2124 = To Double Precision Float(number=w3603) -> (double precision float=w3617:dbl)
                n2125 = Build Array(w3614, w3619, w3625, w3624, w3623, 0.0 ("f")) -> (w3622:dbl[])
                n2126 = Build Array(w3617, w3608, w3607, w3606, w3605) -> (w3615:dbl[])
                n2127 = Select(t=u32 4000000000, s=w3613, f="N sets to save") -> (s? t:f=w3611:u32)
                n2128 = Build Array (concatenate)(w3622, w3621, w3615) -> (w3620:dbl[])
              }
              frame 2 {
                w3636 = 0.0 ("f")
                w3633 = FALSE ("Save APD Data\nwith Trap Data")
                # "calibration"
                n2129 = Boolean To (0,1)(Boolean=w3633) -> (0, 1=w3638:i16)
                n2130 = To Double Precision Float(number=w3638) -> (double precision float=w3637:dbl)
                n2131 = Build Array(w3637, w3636, w3636, w3636, w3636) -> (w3635:dbl[])
                n2132 = Build Array(w3634, w3639, w3639, w3646, w3645, 1.0 ("t")) -> (w3643:dbl[])
                n2133 = Build Array (concatenate)(w3643, w3642, w3635) -> (w3641:dbl[])
                "Calibrating Trap..." <- TRUE ("Calibrating...")
              }
              frame 4 {
                w3653 = 0.0 ("f")
                # "write file header for a trap \nraster scan"
                # "scan dir (x/y = 0/1)"
                # "cycles/step"
                # "n scans (f/b)"
                # "steps"
                # "freq. range"
                # "AOD raster scan"
                n2134 = local read "Number of F/B Scans (AOD)"() -> (w3660:u16)
                n2135 = local read "Cycles/step (AOD)"() -> (w3662:u64)
                n2136 = local read "Scan Range (MHz)"() -> (w3665:dbl)
                n2137 = local read "Scan steps (AOD)"() -> (w3664:u64)
                n2138 = local read "Scan BD"() -> (w3672:bool)
                n2139 = local read "Save ave N"() -> (w3677:dbl)
                n2140 = Boolean To (0,1)(Boolean=w3672) -> (0, 1=w3671:i16)
                n2141 = To Double Precision Float(number=w3660) -> (double precision float=w3659:dbl)
                n2142 = To Double Precision Float(number=w3664) -> (double precision float=w3663:dbl)
                n2143 = To Double Precision Float(number=w3662) -> (double precision float=w3661:dbl)
                n2144 = To Double Precision Float(number=w3671) -> (double precision float=w3670:dbl)
                n2145 = Multiply(x=w3677, y=w3655) -> (x*y=w3676:dbl)
                n2146 = To Double Precision Float(number=w3648) -> (double precision float=w3654:dbl)
                n2147 = Build Array(w3654, w3653, w3653, w3653, w3653) -> (w3651:dbl[])
                n2148 = local read "N sets should be saved"() -> (w3657:dbl)
                n2149 = Build Array(w3670, w3665, w3663, w3661, w3659) -> (w3667:dbl[])
                n2150 = Build Array(w3650, w3655, w3676, w3675, w3674, 2.0 ("t")) -> (w3669:dbl[])
                n2151 = Round Toward +Infinity(x=w3657) -> (ceil(x): smallest int >= x=w3658:dbl)
                n2152 = Build Array (concatenate)(w3669, w3668, w3651, w3667) -> (w3666:dbl[])
                n2153 = To Unsigned Long Integer(number=w3658) -> (unsigned 32bit integer=w3656:u32)
              }
              frame 8 {
                w3686 = 0.0 ("f")
                # "MCL raster scan"
                n2154 = local read "Number of scans (MCL)"() -> (w3681:u64)
                n2155 = local read "Scan lines (y)"() -> (w3680:u64)
                n2156 = local read "2D or 1D Scan"() -> (w3683:bool)
                n2157 = local read "Scan Range (V)\n(of steps)"() -> (w3702:dbl)
                n2158 = local read "Fast Scan Dir"() -> (w3709:bool)
                n2159 = local read "Cycles/step (MCL)"() -> (w3699:u64)
                n2160 = local read "Scan steps (MCL)"() -> (w3701:u64)
                n2161 = Select(t=w3680, s=w3683, f=w3681) -> (s? t:f=w3682:u64)
                n2162 = Boolean To (0,1)(Boolean=w3683) -> (0, 1=w3685:i16)
                n2163 = local read "Save ave N"() -> (w3714:dbl)
                n2164 = local read "Initial X"() -> (w3688:dbl)
                n2165 = local read "Initial Y"() -> (w3687:dbl)
                n2166 = To Double Precision Float(number=w3685) -> (double precision float=w3684:dbl)
                n2167 = Boolean To (0,1)(Boolean=w3709) -> (0, 1=w3708:i16)
                n2168 = To Double Precision Float(number=w3682) -> (double precision float=w3697:dbl)
                n2169 = To Double Precision Float(number=w3701) -> (double precision float=w3700:dbl)
                n2170 = To Double Precision Float(number=w3699) -> (double precision float=w3698:dbl)
                n2171 = To Double Precision Float(number=w3708) -> (double precision float=w3707:dbl)
                n2172 = Multiply(x=w3714, y=w3693) -> (x*y=w3713:dbl)
                n2173 = To Double Precision Float(number=w3678) -> (double precision float=w3692:dbl)
                n2174 = local read "N sets should be saved (MCL)"() -> (w3695:dbl)
                n2175 = Build Array(w3692, w3684, w3686, w3686, w3686) -> (w3690:dbl[])
                n2176 = Build Array(w3707, w3702, w3700, w3698, w3697, w3688, w3687) -> (w3704:dbl[])
                n2177 = Build Array(w3689, w3693, w3713, w3712, w3711, 3.0 ("t")) -> (w3706:dbl[])
                n2178 = Round Toward +Infinity(x=w3695) -> (ceil(x): smallest int >= x=w3696:dbl)
                n2179 = Build Array (concatenate)(w3706, w3705, w3690, w3704) -> (w3703:dbl[])
                n2180 = To Unsigned Long Integer(number=w3696) -> (unsigned 32bit integer=w3694:u32)
              }
            }
            n2181 = local read "Index"() -> (w3553:dbl)
            n2182 = call "Create new save file.vi"("Insert"="", "Ext"=".dat", "Index In"=w3553) -> ("Path Out"=w3512:path, "Index Out"=w3525:dbl)
            n2183 = local write "Save file name"(w3512) -> ()
            n2184 = local write "Index"(w3525) -> ()
            n2185 = local write "Save index"(w3525) -> ()
            n2186 = Array Size(array=w3536) -> (size(s)=w3537:i32)
            n2187 = Open/Create/Replace File(file path (use dialog)=w3512, operation (0:open)=T24."create", access (0:read/write)=enum16{"read/write", "read-only", "write-only"}."write-only") -> (refnum out=w3550:refnum<file>)  [unwired: 1 in, 4 out]
            n2188 = local write "Saving..."(TRUE ("Saving...")) -> ()
            n2189 = To Double Precision Float(number=w3537) -> (double precision float=w3535:dbl)
            n2190 = String Length(string="Comment (data description)") -> (length=w3533:i32)
            n2191 = To Double Precision Float(number=w3533) -> (double precision float=w3532:dbl)
            n2192 = Deny Access(7:w3550) -> (3:w3549:refnum<file>)  [unwired: 1 in, 2 out]
            n2193 = Build Array (concatenate)(w3535, w3536, w3532) -> (w3534:dbl[])
            n2194 = case "If fluorescence data to be saved" shown="True" w3523 {
              tunnel: w3512 -> [_ w3602]
              tunnel: [refnum<k0> refnum w3582] -> w3524
              frame False {
              }
              frame True {
                w3581 = 0.0
                n2195 = local read "APD Integration Time (s)"() -> (w3587:dbl)
                n2196 = local read "N APD Samp/step"() -> (w3580:dbl)
                n2197 = Path To String(path=w3602) -> (string=w3601:string)
                n2198 = String Length(string=w3601) -> (length=w3600:i32)
                n2199 = Subtract(x=w3600, y=4) -> (x-y=w3598:i32)
                n2200 = String Subset(string=w3601, length (rest)=w3598) -> (substring=w3597:string)  [unwired: 1 out]
                n2201 = Build Array(w3587, w3580, w3581, w3581, w3581, w3581, w3581, w3581) -> (w3584:dbl[])
                n2202 = Concatenate Strings(w3597, "_fl.dat" ("string")) -> (w3595:string)
                n2203 = Array Size(array=w3584) -> (size(s)=w3586:i32)
                n2204 = String To Path(string=w3595) -> (path=w3591:path)
                n2205 = Open/Create/Replace File(file path (use dialog)=w3591, operation (0:open)=T24."create", access (0:read/write)=enum16{"read/write", "read-only", "write-only"}."write-only") -> (refnum out=w3592:refnum<file>)  [unwired: 1 in, 4 out]
                n2206 = Deny Access(7:w3592) -> (3:w3588:refnum<file>)  [unwired: 1 in, 2 out]
                n2207 = To Double Precision Float(number=w3586) -> (double precision float=w3585:dbl)
                n2208 = Build Array (concatenate)(w3585, w3584) -> (w3583:dbl[])
                n2209 = Write to Binary File(file (use dialog)=w3588, data=w3583, 5:FALSE ("prepend array or string size? (T)"), 9:T30."big-endian, network order" ("byte order (0:big-endian, network order)")) -> (refnum out=w3582:refnum<file>)  [unwired: 1 in, 3 out]
              }
            }
            n2210 = case shown="True" w3510 {
              tunnel: w3512 -> [_ w3564]
              tunnel: [refnum<k0> refnum w3563] -> w3511
              frame False {
              }
              frame True {
                w3559 = 0.0 ("element")
                n2211 = Path To String(path=w3564) -> (string=w3578:string)
                n2212 = Build Array(w3559, w3559, w3559, w3559, w3559, w3559, w3559, w3559) -> (w3560:dbl[])
                n2213 = String Length(string=w3578) -> (length=w3577:i32)
                n2214 = Subtract(x=w3577, y=4) -> (x-y=w3575:i32)
                n2215 = Array Size(array=w3560) -> (size(s)=w3562:i32)
                n2216 = String Subset(string=w3578, length (rest)=w3575) -> (substring=w3574:string)  [unwired: 1 out]
                n2217 = To Double Precision Float(number=w3562) -> (double precision float=w3561:dbl)
                n2218 = Concatenate Strings(w3574, "_pos.dat" ("string")) -> (w3572:string)
                n2219 = Build Array (concatenate)(w3561, w3560) -> (w3558:dbl[])
                n2220 = String To Path(string=w3572) -> (path=w3568:path)
                n2221 = Open/Create/Replace File(file path (use dialog)=w3568, operation (0:open)=T24."create", access (0:read/write)=enum16{"read/write", "read-only", "write-only"}."write-only") -> (refnum out=w3569:refnum<file>)  [unwired: 1 in, 4 out]
                n2222 = Deny Access(7:w3569) -> (3:w3565:refnum<file>)  [unwired: 1 in, 2 out]
                n2223 = Write to Binary File(file (use dialog)=w3565, data=w3558, 5:FALSE ("prepend array or string size? (T)"), 9:T30."big-endian, network order" ("byte order (0:big-endian, network order)")) -> (refnum out=w3563:refnum<file>)  [unwired: 1 in, 3 out]
              }
            }
            n2224 = Write to Binary File(file (use dialog)=w3549, data=w3534, 5:w3530, 9:w3528) -> (refnum out=w3531:refnum<file>)  [unwired: 1 in, 3 out]
            n2225 = Write to Binary File(file (use dialog)=w3531, data="Comment (data description)", 5:w3530, 9:w3528) -> (refnum out=w3527:refnum<file>)  [unwired: 1 in, 3 out]
          }
        }
        n2226 = feedback-in #19(w3470) -> ()
        n2227 = feedback-in #20(w3497) -> ()
        n2228 = feedback-in #21(w3469) -> ()
        n2229 = feedback-in #22(w3480) -> ()
        n2230 = feedback-in #23(w3483) -> ()
        n2231 = feedback-in #24(w3496) -> ()
        n2232 = feedback-in #25(w3486) -> ()
      }
      frame #1 {
        n2233 = local read "Saving..."() -> (w3727:bool)
        n2234 = case shown="True" w3727 {
          tunnel: w3731 -> [_ w3741]
          tunnel: w3730 -> [_ w3755]
          tunnel: w3729 -> [_ w3751]
          tunnel: w3728 -> [_ w3750]
          tunnel: w3726 -> [_ w3749]
          tunnel: w3725 -> [_ w3744]
          tunnel: w3724 -> [_ w3743]
          tunnel: w3723 -> [_ w3742]
          tunnel: w3722 -> [_ w3740]
          tunnel: w3721 -> [_ w3738]
          tunnel: w3720 -> [_ w3737]
          tunnel: w3719 -> [_ w3736]
          tunnel: w3718 -> [_ w3735]
          tunnel: w3717 -> [_ w3734]
          tunnel: w3716 -> [_ w3733]
          tunnel: w3715 -> [_ w3732]
          frame False {
          }
          frame True {
            n2235 = Multiply(x=w3741, y=w3740) -> (x*y=→"Time (s)":dbl)
            n2236 = Less Or Equal?(x=w3741, y=w3749) -> (x <= y?=w3753:bool)
            n2237 = Or(x="Stop Saving", y="Abort save 2") -> (x .or. y?=w3745:bool)
            n2238 = Not(x=w3745) -> (.not. x?=w3754:bool)
            n2239 = And(x=w3753, y=w3754) -> (x .and. y?=w3752:bool)
            n2240 = case shown="True" w3752 {
              tunnel: w3755 -> [w3762 w3830]
              tunnel: [0.0 w3833] -> w3748
              tunnel: w3741 -> [_ w3831]
              tunnel: w3749 -> [_ w3832]
              tunnel: w3751 -> [_ w3827]
              tunnel: w3750 -> [_ _]
              tunnel: w3744 -> [w3760 w3820]
              tunnel: w3743 -> [w3759 w3821]
              tunnel: w3742 -> [_ w3819]
              tunnel: w3738 -> [_ w3818]
              tunnel: w3737 -> [_ w3772]
              tunnel: w3736 -> [_ w3811]
              tunnel: w3735 -> [_ w3789]
              tunnel: w3734 -> [w3757 w3770]
              tunnel: w3733 -> [w3758 w3769]
              tunnel: w3732 -> [_ w3766]
              frame False {
                w3756 = FALSE
                n2241 = Close File(refnum=w3762) -> ()  [unwired: 1 in, 2 out]
                n2242 = case shown="True" w3759 {
                  tunnel: w3760 -> [_ w3764]
                  frame False {
                  }
                  frame True {
                    n2243 = Close File(refnum=w3764) -> ()  [unwired: 1 in, 2 out]
                  }
                }
                n2244 = case shown="True" w3757 {
                  tunnel: w3758 -> [_ w3763]
                  frame False {
                  }
                  frame True {
                    n2245 = Close File(refnum=w3763) -> ()  [unwired: 1 in, 2 out]
                  }
                }
                n2246 = local write "Calibrating Trap..."(w3756) -> ()
                n2247 = call <vilib>:"Beep.vi"() -> ()  [unwired: 3 in, 9 out]
                n2248 = local write "Stop Saving"(w3756) -> ()
                n2249 = property on="Raster Scanning..." class="Bool (strict)"("Val(Sgnl)"=w3756) -> ()  [unwired: 2 in, 2 out]
                "Saving..." <- w3756
              }
              frame True {
                n2250 = local read "Calibrating Trap..."() -> (w3822:bool)
                n2251 = case "Write fl. data" shown="True" w3821 {
                  tunnel: w3820 -> [_ w3856]
                  tunnel: w3819 -> [_ w3855]
                  frame False {
                  }
                  frame True {
                    n2252 = Write to Binary File(file (use dialog)=w3856, data=w3855, 5:FALSE ("prepend array or string size? (T)"), 9:T30."big-endian, network order" ("byte order (0:big-endian, network order)")) -> ()  [unwired: 1 in, 4 out]
                  }
                }
                n2253 = Greater?(x="Save ave N", y=1.0) -> (0:w3825:bool)
                n2254 = Not(x=w3822) -> (.not. x?=w3824:bool)
                n2255 = And(x=w3824, y=w3825) -> (x .and. y?=w3767:bool)
                n2256 = case shown="True" w3767 {
                  tunnel: w3766 -> [w3836 w3847]
                  tunnel: [w3836 w3839] -> w3765
                  tunnel: "Save ave N" -> [_ w3840]
                  frame False {
                  }
                  frame True {
                    w3837 = 2 ("dimension size")
                    n2257 = Array Size(array=w3847) -> (size(s)=w3841:i32)
                    n2258 = Divide(x=w3841, y=w3837) -> (x/y=w3845:dbl)
                    n2259 = Reshape Array(w3847, w3845, w3837) -> (w3846:u64[][])
                    n2260 = Transpose 2D Array(2D array=w3846) -> (transposed array=w3844:u64[][])
                    n2261 = for {
                      tunnel: w3844 -> [w3849] mode=indexing
                      tunnel: [w3848] -> w3838 mode=indexing
                      tunnel: w3840 -> [w3850]
                      workers-P: _ -> [_]
                      n2262 = call "downsample 1D array - U64.vi"("Ave N"=w3850, "Array In"=w3849) -> ("Array Out"=w3848:u64[])  [unwired: 1 in]
                    }
                    n2263 = Transpose 2D Array(2D array=w3838) -> (transposed array=w3843:u64[][])
                    n2264 = Divide(x=w3841, y=w3840) -> (x/y=w3842:dbl)
                    n2265 = Reshape Array(w3843, w3842) -> (w3839:u64[])
                  }
                }
                n2266 = case shown="True" w3767 {
                  tunnel: w3827 -> [w3859 w3871]
                  tunnel: [w3859 w3863] -> w3823
                  tunnel: "Save ave N" -> [_ w3864]
                  tunnel: w3818 -> [_ w3862]
                  frame False {
                    # "don't downsample data for trap calibration"
                  }
                  frame True {
                    n2267 = Array Size(array=w3871) -> (size(s)=w3865:i32)
                    n2268 = Array Size(array=w3862) -> (size(s)=w3861:i32)
                    n2269 = Divide(x=w3865, y=w3861) -> (x/y=w3869:dbl)
                    n2270 = Reshape Array(w3871, w3869, w3861) -> (w3870:i16[][])
                    n2271 = Transpose 2D Array(2D array=w3870) -> (transposed array=w3868:i16[][])
                    n2272 = for {
                      tunnel: w3868 -> [w3874] mode=indexing
                      tunnel: [w3873] -> w3860 mode=indexing
                      tunnel: w3864 -> [w3872]
                      workers-P: _ -> [_]
                      n2273 = call "downsample 1D array - I16.vi"("Ave N"=w3872, "Array In"=w3874) -> ("Array Out"=w3873:i16[])  [unwired: 1 out]
                    }
                    n2274 = Transpose 2D Array(2D array=w3860) -> (transposed array=w3867:i16[][])
                    n2275 = Divide(x=w3865, y=w3864) -> (x/y=w3866:dbl)
                    n2276 = Reshape Array(w3867, w3866) -> (w3863:i16[])
                  }
                }
                n2277 = Index Array(array=w3789, index=1) -> (element=w3792:waveform(dbl))
                n2278 = Index Array(array=w3789, index=0) -> (element=w3794:waveform(dbl))
                n2279 = Unbundle By Name(w3792) -> ("Y"=w3796:dbl[])
                n2280 = Unbundle By Name(w3794) -> ("Y"=w3804:dbl[])
                n2281 = case "Write trap pos. data" shown="True" w3770 {
                  tunnel: w3769 -> [_ w3852]
                  tunnel: w3765 -> [_ w3851]
                  frame False {
                  }
                  frame True {
                    n2282 = Write to Binary File(file (use dialog)=w3852, data=w3851, 5:FALSE ("prepend array or string size? (T)"), 9:T30."big-endian, network order" ("byte order (0:big-endian, network order)")) -> ()  [unwired: 1 in, 4 out]
                  }
                }
                n2283 = Write to Binary File(file (use dialog)=w3830, data=w3823, 5:FALSE ("prepend array or string size? (T)"), 9:T30."big-endian, network order" ("byte order (0:big-endian, network order)")) -> ()  [unwired: 1 in, 4 out]
                n2284 = feedback #26(w3796) -> (w3798:dbl[])
                n2285 = Build Array (concatenate)(w3798, w3796) -> (w3797:dbl[])
                n2286 = Select(t=w3796, s=w3772, f=w3797) -> (s? t:f=w3782:dbl[])
                n2287 = feedback-in #26(w3782) -> ()
                n2288 = feedback #27(w3804) -> (w3817:dbl[])
                n2289 = Build Array (concatenate)(w3817, w3804) -> (w3816:dbl[])
                n2290 = Select(t=w3804, s=w3772, f=w3816) -> (s? t:f=w3791:dbl[])
                n2291 = feedback-in #27(w3791) -> ()
                n2292 = Divide(x=w3831, y=w3832) -> (x/y=w3834:dbl)
                n2293 = Multiply(x=w3834, y=100.0) -> (x*y=w3833:dbl)
                n2294 = Build Array(w3791, w3782) -> (→"Saved APD":dbl[][])
                n2295 = Array Size(array=w3791) -> (size(s)=w3809:i32)
                n2296 = Unbundle By Name(w3811) -> ("Y"=w3815:dbl[])
                n2297 = Subtract(x=w3809, y="N pts to average") -> (x-y=w3785:i32)
                n2298 = Multiply(x="N pts to average", y=u16 2) -> (x*y=w3786:u16)
                n2299 = Subtract(x=w3809, y=w3786) -> (x-y=w3784:i32)
                n2300 = feedback #28(w3815) -> (w3814:dbl[])
                n2301 = Build Array (concatenate)(w3814, w3815) -> (w3813:dbl[])
                n2302 = Select(t=w3815, s=w3772, f=w3813) -> (s? t:f=w3812:dbl[])
                "Trap Delta Graph" <- w3812
                n2303 = feedback-in #28(w3812) -> ()
                n2304 = Array Subset(array=w3791, index=w3785, length="N pts to average") -> (w3808:dbl[])
                n2305 = Array Subset(array=w3791, index=w3784, length="N pts to average") -> (w3807:dbl[])
                n2306 = Array Subset(array=w3782, index=w3785, length="N pts to average") -> (w3788:dbl[])
                n2307 = Array Subset(array=w3782, index=w3784, length="N pts to average") -> (w3787:dbl[])
                n2308 = call-poly <vilib>:"Mean.vi"("X"=w3808) -> ("mean"=w3806:dbl)  [unwired: 1 out]
                n2309 = call-poly <vilib>:"Mean.vi"("X"=w3788) -> ("mean"=w3781:dbl)  [unwired: 1 out]
                n2310 = call-poly <vilib>:"Mean.vi"("X"=w3807) -> ("mean"=w3805:dbl)  [unwired: 1 out]
